vi "mqttRXsubscriptionEvent.vi"(2 "function":T2=enum."getEventRef", 7 "data":T1, 11 "error in (no error)":errorcluster) -> (4 "subscriptionData":refnum<user-event>, 15 "error out":errorcluster)   [LabVIEW 2022 SP3]
uses:
  mqttRXsubscriptionEventFunction.ctl
  mqttRXsubscriptionEventData.ctl
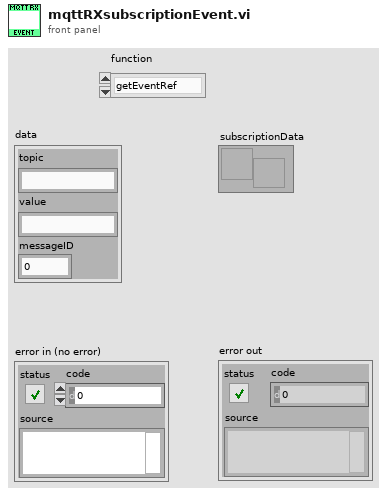
[diagram p1: front panel]
types:
  T1 = typedef "mqttRXsubscriptionEventData.ctl" = cluster{"topic":string, "value":string, "messageID":u16}
  T2 = typedef "mqttRXsubscriptionEventFunction.ctl" = enum16{"init", "deinit", "getEventRef", "event"}
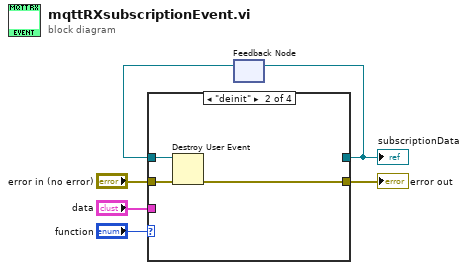
[diagram p0: block diagram]
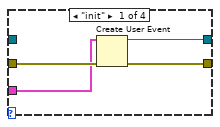
[diagram p2: hidden frame]
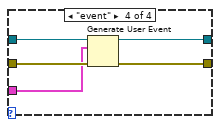
[diagram p4: hidden frame]
diagram:
  n1 = feedback #1() -> (w5:refnum<user-event>)  [unwired: 1 in]
  n2 = case shown="\"deinit\"" "function" {
    tunnel: "data" -> [w7 _ _ w16]
    tunnel: [w10 _ w15 w18] -> w2
    tunnel: w5 -> [_ w13 w15 w19]
    tunnel: "error in (no error)" -> [w9 w12 w14 w20]
    tunnel: [w8 w11 w14 w17] -> w3
    frame "init" {
      n3 = Create User Event(user event datatype=w7, error in=w9) -> (user event=w10:refnum<user-event>, error out=w8:errorcluster)
    }
    frame "deinit" {
      n4 = Destroy User Event(user event=w13, error in=w12) -> (error out=w11:errorcluster)
    }
    frame "getEventRef" {
    }
    frame "event" {
      n5 = Generate User Event(user event=w19, event data cluster=w16, error in=w20) -> (user event out=w18:refnum<user-event>, error out=w17:errorcluster)  [unwired: 1 in]
    }
  }
  "error out" <- w3
  "subscriptionData" <- w2
  n6 = feedback-in #1(w2) -> ()
